vi "Dual DM Control - MAIN V1.vi"() -> ()   [LabVIEW 2014]
uses:
  DMControl_V3.ctl
panel:
  in  "Top Mirror":T1 {"Modes"."Amplititude" step=0.05}
  in  "Bottom Mirror":T1 {"Modes"."Amplititude" step=0.05}
  in  "Stop":bool
  out "Top Mirror":dbl[][](graph)
  out "Bottom Mirror":dbl[][](graph)
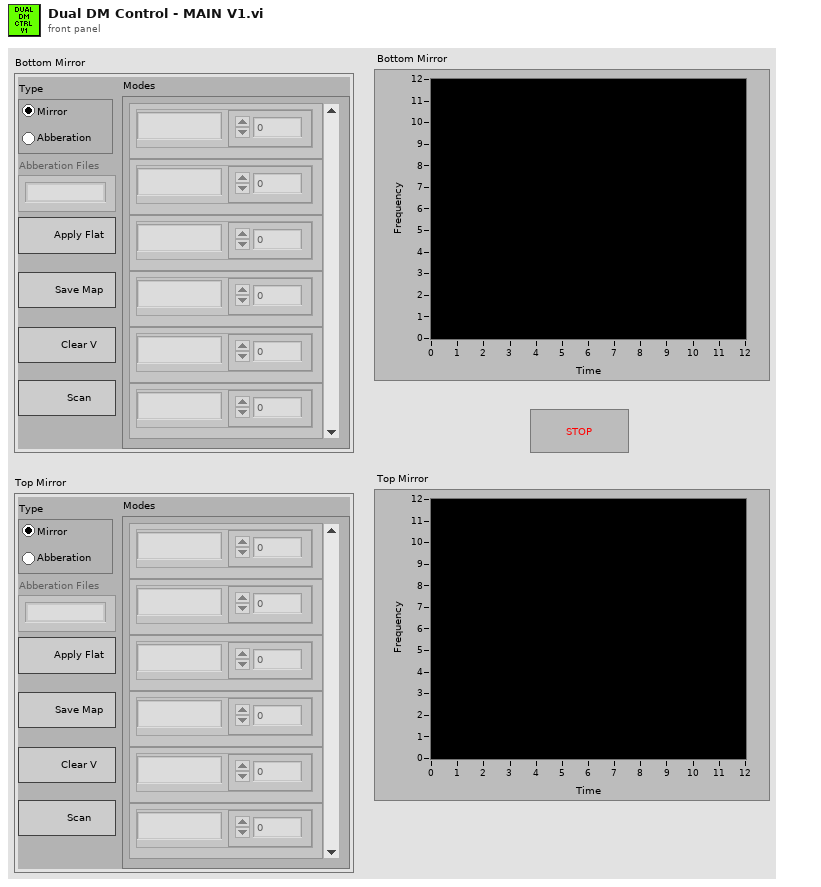
[diagram p1: front panel]
types:
  T1 = typedef "DMControl_V3.ctl" = cluster{"Type":enum32{"Mirror", "Abberation"}, "Modes":cluster{"Mode":string, "Amplititude":dbl}[], "Apply Flat":bool, "Save Map":bool, "Clear Voltage":bool, "Abberation Files":u16, "Scan ":bool}
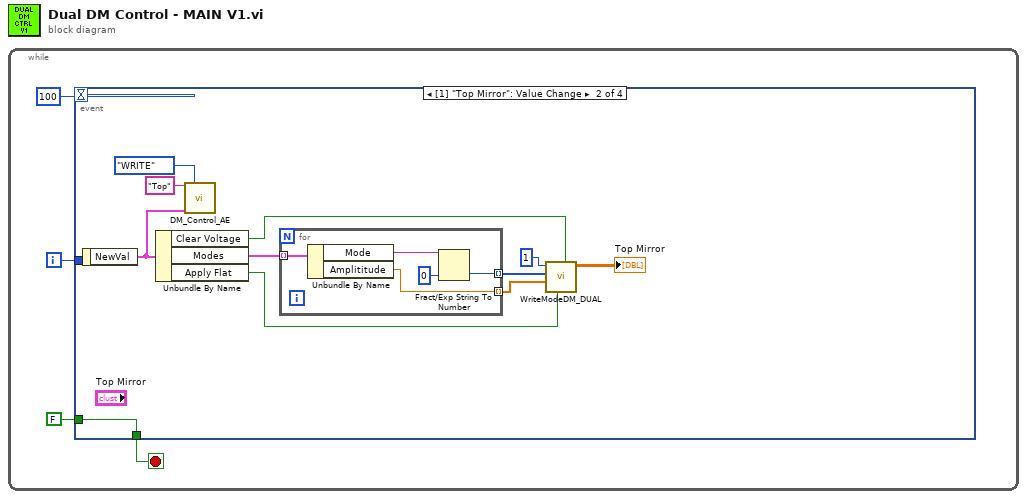
[diagram p0: block diagram]
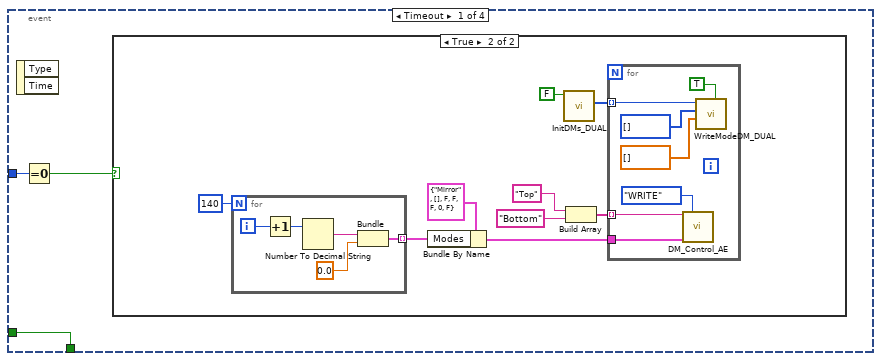
[diagram p2: hidden frame]
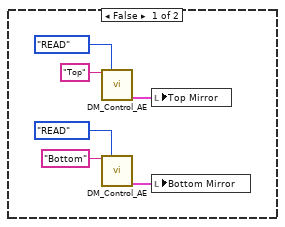
[diagram p3: hidden frame]
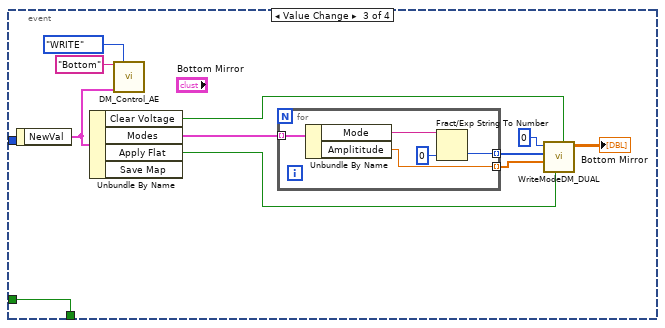
[diagram p4: hidden frame]
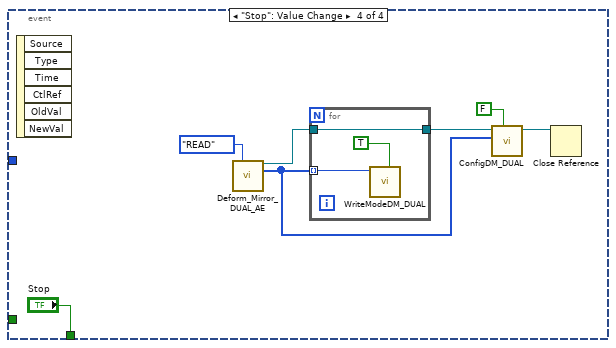
[diagram p5: hidden frame]
diagram:
  n1 = while {
    i -> [w1]
    stop <- w3 stop-if-true
    n2 = event shown="[1] \"Top Mirror\": Value Change" {
      selector: _ -> [_ _ _ _]
      dyn-events: _ -> [_ _ _ _]
      timeout: 100 -> [_ _ _ _]
      tunnel: [w5 w45 w61 "Stop"] -> w3
      tunnel: FALSE -> [w5 w45 w61 _]
      tunnel: w1 -> [w7 _ _ _]
      event Timeout {
        n3 = event-data() -> ()  [unwired: 1 in, 2 out]
        n4 = Equal To 0?(x=w7) -> (x = 0?=w6:bool)
        n5 = case shown="True" w6 {
          frame False {
            n6 = call "DM_Control_AE.vi"("Mirror ID"="Top", "Action"=enum16{"WRITE", "READ"}."READ") -> ("Mirror Control OUT"=w9:T1)  [unwired: 12 in, 1 out]
            n7 = call "DM_Control_AE.vi"("Mirror ID"="Bottom", "Action"=enum16{"WRITE", "READ"}."READ") -> ("Mirror Control OUT"=w8:T1)  [unwired: 12 in, 1 out]
            n8 = local write "Top Mirror"(w9) -> ()
            n9 = local write "Bottom Mirror"(w8) -> ()
          }
          frame True {
            n10 = for {
              N: 140 -> [_]
              tunnel: [w23] -> w21 mode=indexing
              i -> [w27]
              n11 = Increment(x=w27) -> (x+1=w26:i32)
              n12 = Number To Decimal String(number=w26) -> (decimal integer string=w25:string)  [unwired: 1 in]
              n13 = Bundle(w25, 0.0) -> (w23:cluster{string, dbl})  [unwired: 1 in]
            }
            n14 = Bundle By Name(cluster=T1 {"Type"=enum."Mirror", "Modes"=[], "Apply Flat"=FALSE, "Save Map"=FALSE, "Clear Voltage"=FALSE, "Abberation Files"=0, "Scan "=FALSE} ("Bottom Mirror"), "Modes"=w21) -> (w22:T1)
            n15 = call "InitDMs_DUAL.vi"("BM Flats"=FALSE) -> ("IDs"=w18:i32[])  [unwired: 9 in, 1 out]
            n16 = Build Array("Top" ("Mirror ID"), "Bottom" ("Mirror ID")) -> (w16:string[])
            n17 = for {
              tunnel: w18 -> [w34] mode=indexing
              tunnel: w16 -> [w29] mode=indexing
              tunnel: w22 -> [w28]
              n18 = call "DM_Control_AE.vi"("Mirror ID"=w29, "Action"=enum16{"WRITE", "READ"}."WRITE", "Mirror Control IN"=w28) -> ()  [unwired: 11 in, 2 out]
              n19 = call "WriteModeDM_DUAL.vi"("Clear DM Voltage"=TRUE, "Amplitudes"=dbl[] [], "Modes"=i32[] [], "Device"=w34) -> ()  [unwired: 6 in, 2 out]
            }
          }
        }
      }
      event Value Change {
        n20 = event-data() -> ("NewVal"=w35:T1)  [unwired: 1 in]
        n21 = Unbundle By Name(w35) -> ("Clear Voltage"=w40:bool, "Modes"=w43:cluster{"Mode":string, "Amplititude":dbl}[], "Apply Flat"=w39:bool)
        n22 = call "DM_Control_AE.vi"("Mirror ID"="Top", "Action"=enum16{"WRITE", "READ"}."WRITE", "Mirror Control IN"=w35) -> ()  [unwired: 11 in, 2 out]
        n23 = for {
          tunnel: w43 -> [w50] mode=indexing
          tunnel: [w47] -> w42 mode=indexing
          tunnel: [w46] -> w41 mode=indexing
          n24 = Unbundle By Name(w50) -> ("Mode"=w48:string, "Amplititude"=w46:dbl)
          n25 = Fract/Exp String To Number(string=w48, default (0 dbl)=0) -> (number=w47:i32)  [unwired: 2 in, 1 out]
        }
        n26 = call "WriteModeDM_DUAL.vi"("Clear DM Voltage"=w40, "Flat File ON"=w39, "Amplitudes"=w41, "Modes"=w42, "Device"=1) -> ("Voltage Map"=→"Top Mirror":dbl[][])  [unwired: 5 in, 1 out]
      }
      event Value Change {
        n27 = event-data() -> ("NewVal"=w51:T1)  [unwired: 1 in]
        n28 = Unbundle By Name(w51) -> ("Clear Voltage"=w56:bool, "Modes"=w59:cluster{"Mode":string, "Amplititude":dbl}[], "Apply Flat"=w55:bool)  [unwired: 1 out]
        n29 = call "DM_Control_AE.vi"("Mirror ID"="Bottom", "Action"=enum16{"WRITE", "READ"}."WRITE", "Mirror Control IN"=w51) -> ()  [unwired: 11 in, 2 out]
        n30 = for {
          tunnel: w59 -> [w66] mode=indexing
          tunnel: [w63] -> w58 mode=indexing
          tunnel: [w62] -> w57 mode=indexing
          n31 = Unbundle By Name(w66) -> ("Mode"=w64:string, "Amplititude"=w62:dbl)
          n32 = Fract/Exp String To Number(string=w64, default (0 dbl)=0) -> (number=w63:i32)  [unwired: 2 in, 1 out]
        }
        n33 = call "WriteModeDM_DUAL.vi"("Clear DM Voltage"=w56, "Flat File ON"=w55, "Amplitudes"=w57, "Modes"=w58, "Device"=0) -> ("Voltage Map"=→"Bottom Mirror":dbl[][])  [unwired: 5 in, 1 out]
      }
      event "Stop": Value Change {
        n34 = event-data() -> ()  [unwired: 1 in, 6 out]
        n35 = call "Deform_Mirror_DUAL_AE.vi"("Action"=enum16{"WRITE", "READ"}."READ") -> ("Refnum Out"=w71:refnum<k7>, "IDs Out"=w68:i32[])  [unwired: 10 in, 3 out]
        n36 = for {
          tunnel: w68 -> [w76] mode=indexing
          tunnel: w71 -> [w74]
          tunnel: [w74] -> w69
          n37 = call "WriteModeDM_DUAL.vi"("Clear DM Voltage"=TRUE, "Device"=w76) -> ()  [unwired: 8 in, 2 out]
        }
        n38 = call "ConfigDM_DUAL.vi"("High Voltage"=FALSE, "Dev IDs"=w68, "Automation Refnum in"=w69) -> ("Automation Refnum out"=w67:refnum<k7>)  [unwired: 7 in, 1 out]
        n39 = Close Reference(reference=w67) -> ()  [unwired: 1 in, 1 out]
      }
    }
  }
